vi "testAESEncryptDecrypt-CBC-256-ManualIV.vi"(8 "error in (no error)":errorcluster, 11 "TestCase in":refnum<class "TestAES.lvclass">) -> (0 "error out":errorcluster, 3 "TestCase out":refnum<class "TestAES.lvclass">)   [LabVIEW 2021, in "TestAES.lvclass"]
uses:
  TestAES.lvclass
  C:/Program Files (x86)/National Instruments/LabVIEW 2021/vi.lib/addons/_JKI Toolkits/VI Tester/TestCase.llb/TestCase.lvclass
  <vilib>/addons/_JKI Toolkits/VI Tester/TestCase.llb/TestCase.lvclass
  <vilib>/Wiresmith Technology/VITAC (VI Tester Advanced Comparisons)/VITAC.lvlib
  Source Code/Symmetric Encryption/dotNET Crypto Symmetric Encryption.lvlib
panel:
  out "Encrypted data out":u8[](array[numeric])
  out "IV out":u8[](array[numeric])
  out "Plaintext in (hex)":string="Hello, World!"
  out "Key (hex)":string="01234567890"
  out "Expected plaintext (hex)":string
  out "Actual plaintext out (hex)":string
  out "Expected plaintext":string
  out "Plaintext in":string="Hello, World!"
  out "Actual plaintext out":string
  out "Key":string="01234567890"
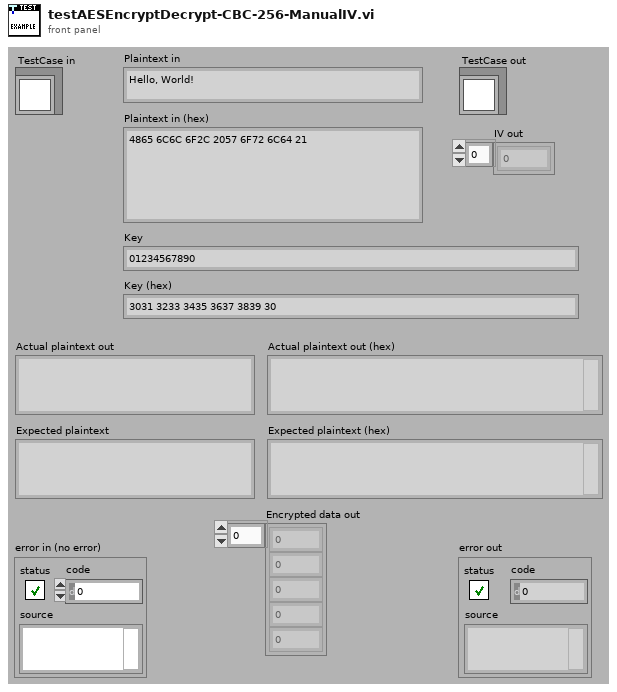
[diagram p1: front panel]
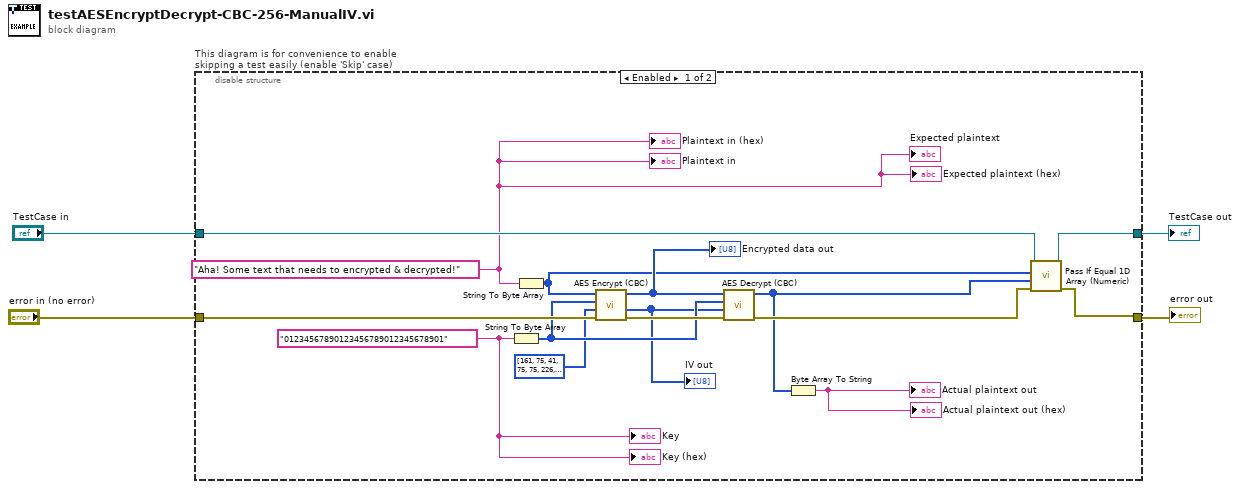
[diagram p0: block diagram]
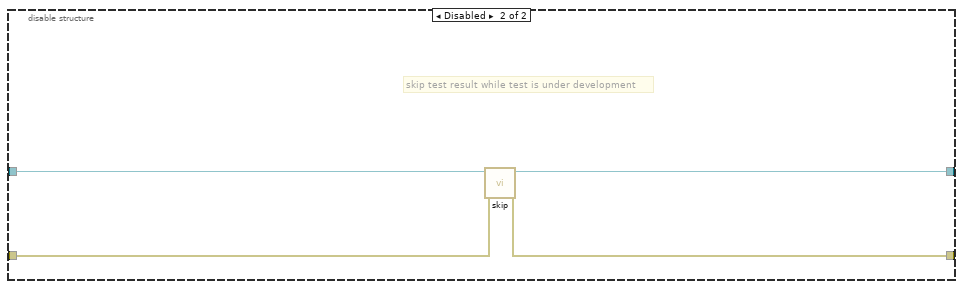
[diagram p2: hidden frame]
diagram:
  n1 = disable-structure "This diagram is for convenience to enable skipping a test easily (enable 'Skip' case)" shown="Enabled" {
    disable-tunnel: "TestCase in" -> [w19 w23]
    disable-tunnel: [w18 w21] -> w1
    disable-tunnel: [w17 w22] -> w3
    disable-tunnel: "error in (no error)" -> [w16 w20]
    frame Enabled {
      w12 = "01234567890123456789012345678901" ("Key")
      w8 = "Aha! Some text that needs to encrypted & decrypted!" ("Plaintext in")
      n2 = String To Byte Array(string=w12) -> (unsigned byte array=w11:u8[])
      n3 = String To Byte Array(string=w8) -> (unsigned byte array=w7:u8[])
      n4 = call "AES Encrypt (CBC).vi"("error in (no error)"=w16, "IV"=u8[] [161, 75, 41, 75, 75, 226, 165, 48, 194, 72, 167, 18, 180, 152, 94, 91] ("IV out"), "Key"=w11, "Raw data in"=w7) -> ("error out"=w15:errorcluster, "IV out"=w6:u8[], "Encrypted data out"=w13:u8[])  [unwired: 5 in]
      "IV out" <- w6
      "Encrypted data out" <- w13
      n5 = call "AES Decrypt (CBC).vi"("error in (no error)"=w15, "IV"=w6, "Key"=w11, "Encrypted data in"=w13) -> ("error out"=w14:errorcluster, "Raw data out"=w9:u8[])  [unwired: 6 in]
      n6 = Byte Array To String(unsigned byte array=w9) -> (string=→"Actual plaintext out" →"Actual plaintext out (hex)":string)
      n7 = call <vilib>:"Pass If Equal 1D Array (Numeric).vi"("error in (no error)"=w14, "actual"=w9, "expected"=w7, "TestCase in"=w19) -> ("error out"=w17:errorcluster, "TestCase out"=w18:refnum<class "TestAES.lvclass">)  [unwired: 6 in]
      "Key" <- w12
      "Plaintext in" <- w8
      "Expected plaintext" <- w8
      "Expected plaintext (hex)" <- w8
      "Key (hex)" <- w12
      "Plaintext in (hex)" <- w8
    }
    frame Disabled {
      # "skip test result while test is under development"
      n8 = call <vilib>:"skip.vi"("error in (no error)"=w20, "TestCase in"=w23) -> ("error out"=w22:errorcluster, "TestCase out"=w21:refnum<class "TestAES.lvclass">)  [unwired: 8 in]
    }
  }
  "error out" <- w3
  "TestCase out" <- w1
